vi "TestBed.vi"() -> ()   [LabVIEW 2014]
uses:
  CntrlRefs.ctl
  Modules/BusClass/Bus.lvclass
  UserEvents/clUserEventDataType.ctl
  Modules/BusClass/Bus.lvclass/Bus.ctl
  Modules/BusClass/Accessors/Write BusNumber.vi
  Modules/BusClass/Accessors/Read Test.vi
  Modules/BusClass/Accessors/Read BusNumber.vi
  <vilib>/Utility/error.llb/Error Cluster From Error Code.vi
  <vilib>/ErrorRing/Error Ring.xnode
  Modules/TestClass/Test.lvclass
  Queue/Queue.lvlib
  <userlib>/NIST/NISTErrorLib/NISTErrorLib.lvlib
  Modules/Sync/SyncModule/SyncModule.lvlib
  Modules/FGen/FgenModule/FgenModule.lvlib
  Modules/Digitizer/DigitizerModule/DigitizerModule.lvlib
  Modules/Sensor/SensorModule/SensorModule.lvlib
  Modules/Analysis/AnalysisModule/AnalysisModule.lvlib
  LV_Ini/Ini_lib.lvlib
panel:
  in  "rngDigitizer":u16(ring)=2 items=["IVI Digitizer", "Analyse Waveforms", "Debug", "Ni DaqMx Digitizer", "PMU Cal", "(obsolete)", "Simulation"]
  in  "rngFgen":u16(ring)=7 items=["DaqMx_Single", "Single_AM", "None", "Agilent IVI FGen", "IVI Dual FGens", "IVI FGen", "Debug", "Pxi6733_Sine", "Pxi6733 Sine Standalone", "PMU Cal", "Test"]
  in  "rngSync":u16(ring)=2 items=["Local", "NI PXI 6682", "6683H class Dyn3", "Debug", "Dyn3 Digitizer", "Dyn3 PMU Cal", "HIL_Sync", "Legacy", "PXI Multi"]
  in  "btnRunScript":bool
  in  "btnClearStatus":bool
  out "Status Log":string
  in  "ModuleList":string[](array[string])=["Sync", "FGen", "Digitizer"]
  in  "btnStop":bool
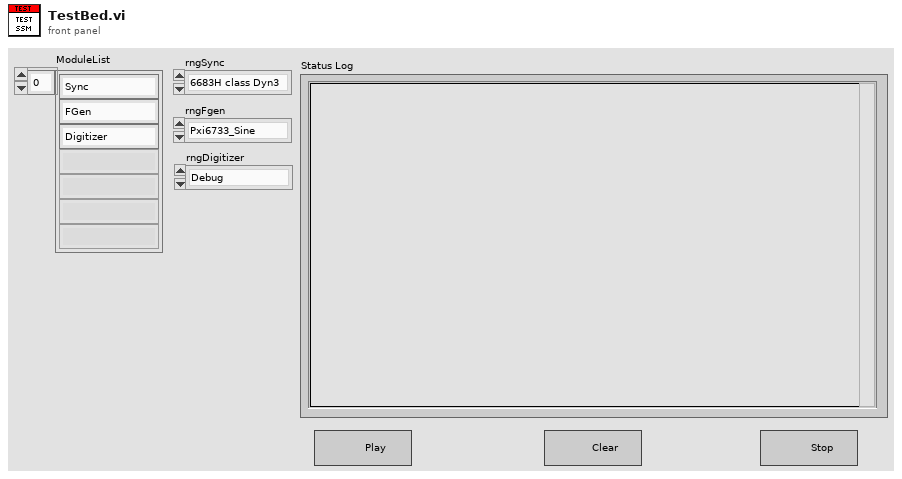
[diagram p1: front panel]
types:
  T1 = typedef "CntrlRefs.ctl" = cluster{"rngFGen":refnum<vi>, "rngDigitizer":refnum<vi>, "rngAnalysis":refnum<vi>, "rngSync":refnum<vi>, "btnHideMods":refnum<vi>, "rngSensor":refnum<vi>}
  T2 = typedef "SyncModule.lvlib/clBroadcastEvents.ctl" = cluster{"DidInit":refnum<user-event>, "StatusUpdate":refnum<user-event>, "ErrorReport":refnum<user-event>, "DidStop":refnum<user-event>, "PathToINI":refnum<user-event>, "TriggerTime":refnum<user-event>, "LockStatus":refnum<user-event>}
  T3 = typedef "FgenModule.lvlib/clBroadcastEvents.ctl" = cluster{"DidInit":refnum<user-event>, "StatusUpdate":refnum<user-event>, "ErrorReport":refnum<user-event>, "DidStop":refnum<user-event>, "PathToINI":refnum<user-event>, "Channels":refnum<user-event>, "Function":refnum<user-event>, "Waveforms":refnum<user-event>, "Triggers":refnum<user-event>}
  T4 = typedef "DigitizerModule.lvlib/clBroadcastEvents.ctl" = cluster{"DidInit":refnum<user-event>, "StatusUpdate":refnum<user-event>, "ErrorReport":refnum<user-event>, "DidStop":refnum<user-event>, "PathToINI":refnum<user-event>, "Channels":refnum<user-event>, "Acq":refnum<user-event>, "Trigger":refnum<user-event>, "Waveforms":refnum<user-event>}
  T5 = typedef "SensorModule.lvlib/clBroadcastEvents.ctl" = cluster{"DidInit":refnum<user-event>, "StatusUpdate":refnum<user-event>, "ErrorReport":refnum<user-event>, "DidStop":refnum<user-event>, "PathToINI":refnum<user-event>, "SensorReport":refnum<user-event>, "SensorConfig":refnum<user-event>}
  T6 = typedef "AnalysisModule.lvlib/clBroadcastEvents.ctl" = cluster{"DidInit":refnum<user-event>, "StatusUpdate":refnum<user-event>, "ErrorReport":refnum<user-event>, "DidStop":refnum<user-event>, "PathToINI":refnum<user-event>, "Config":refnum<user-event>, "ResultReport":refnum<user-event>}
  T7 = typedef "clUserEvents.ctl" = cluster{"StopEvent":refnum<user-event>, "CreateBus":refnum<user-event>, "UpdateEvents":refnum<user-event>}
  T8 = typedef "clUserEventDataType.ctl" = cluster{"Data":variant}
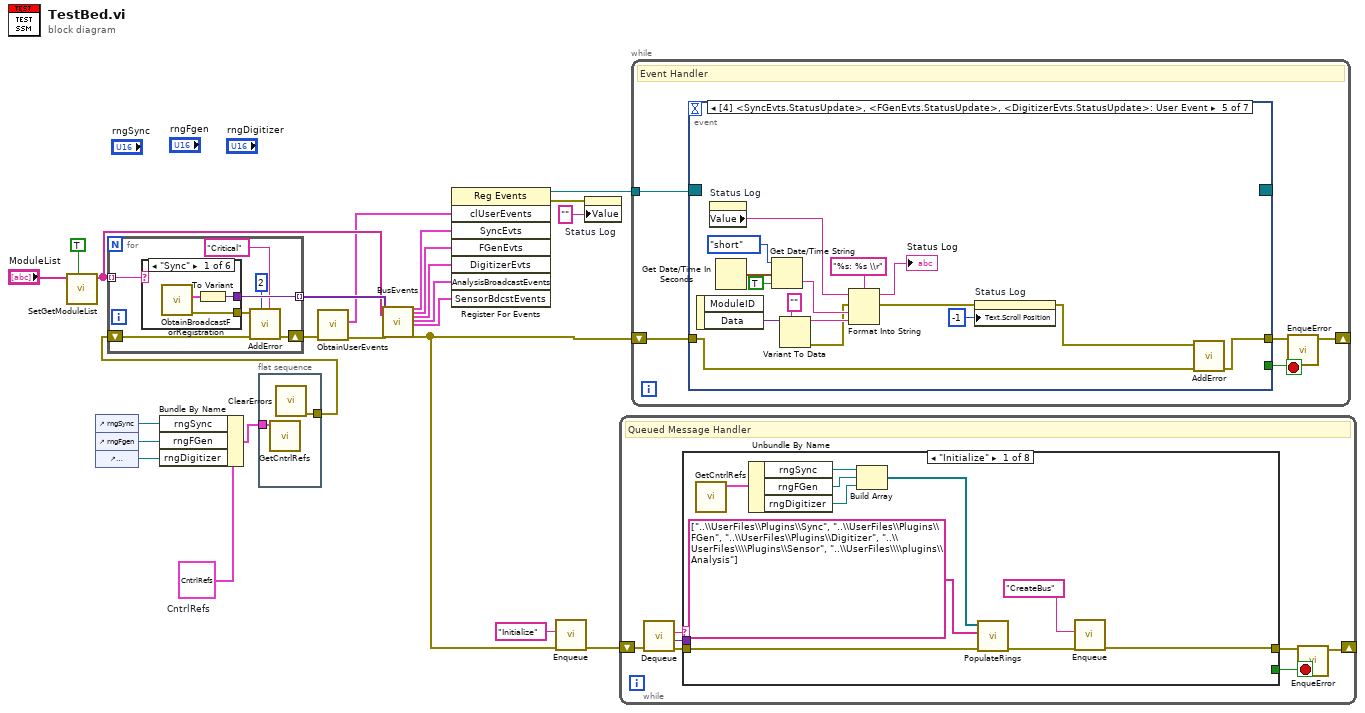
[diagram p0: block diagram]
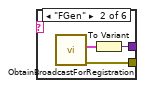
[diagram p2: hidden frame]
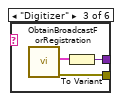
[diagram p3: hidden frame]
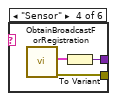
[diagram p4: hidden frame]
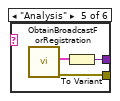
[diagram p5: hidden frame]
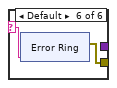
[diagram p6: hidden frame]
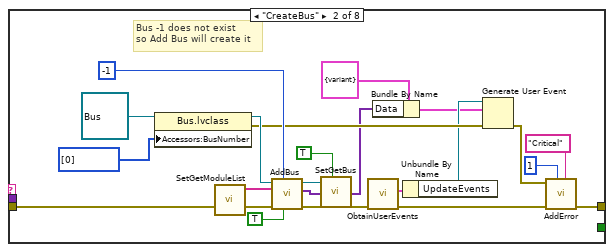
[diagram p7: hidden frame]
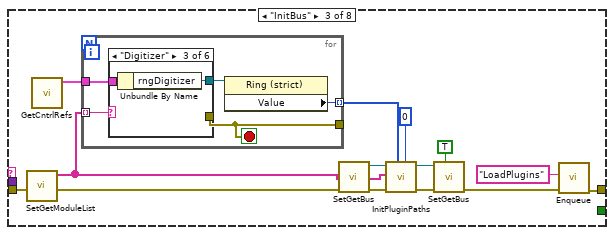
[diagram p8: hidden frame]
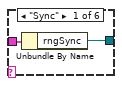
[diagram p9: hidden frame]
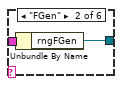
[diagram p10: hidden frame]
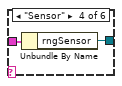
[diagram p11: hidden frame]
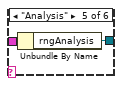
[diagram p12: hidden frame]
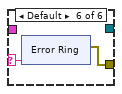
[diagram p13: hidden frame]
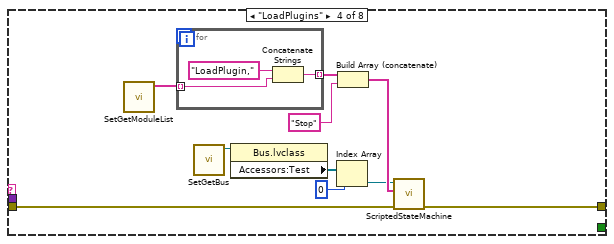
[diagram p14: hidden frame]
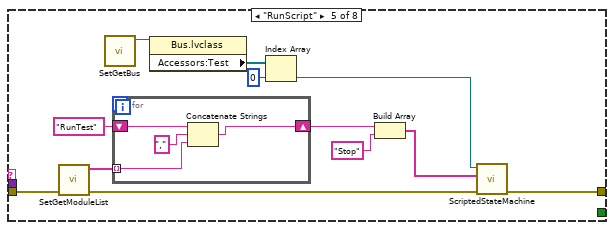
[diagram p15: hidden frame]
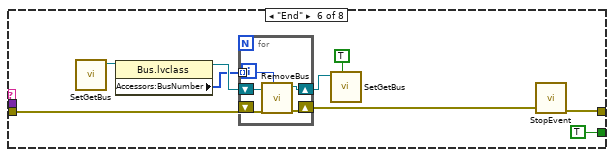
[diagram p16: hidden frame]
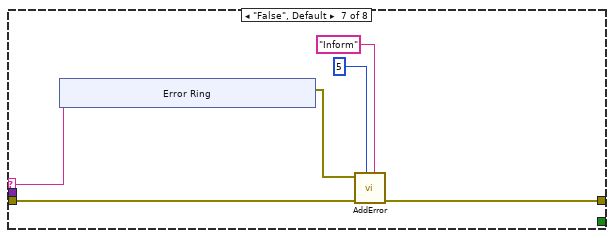
[diagram p17: hidden frame]
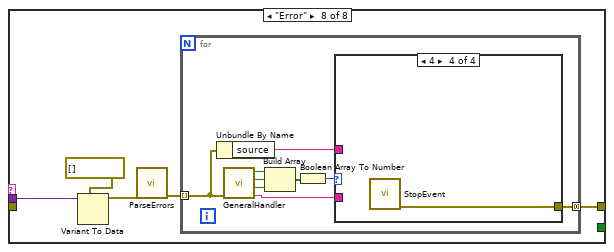
[diagram p18: hidden frame]
diagram:
  w6 = T1 {"rngFGen"=refnum, "rngDigitizer"=refnum, "rngAnalysis"=refnum, "rngSync"=refnum, "btnHideMods"=refnum, "rngSensor"=refnum}  # CntrlRefs
  n1 = call "SetGetModuleList.vi"("Set? (f)"=TRUE, "ModuleList"="ModuleList") -> ("ModuleList"=w19:string[])  [unwired: 9 in]
  n2 = control-ref of="rngSync"() -> (w5:refnum<vi>)
  n3 = control-ref of="rngFgen"() -> (w2:refnum<vi>)
  n4 = control-ref of="rngDigitizer"() -> (w1:refnum<vi>)
  n5 = for {
    shift-right: [w30] -> w9
    shift-left: w3 -> [w29]
    tunnel: [w28] -> w20 mode=indexing
    tunnel: w19 -> [w25] mode=indexing
    n6 = case shown="\"Sync\"" w25 {
      selector: w25 -> [_ _ _ _ _ w47]
      tunnel: [w33 w36 w39 w42 w45 _] -> w28
      tunnel: [w32 w37 w40 w43 w46 w48] -> w31
      frame "Sync" {
        n7 = call "ObtainBroadcastForRegistration.vi"() -> ("error out"=w32:errorcluster, "SyncBroadcastEvents"=w34:T2)  [unwired: 10 in]
        n8 = To Variant(anything=w34) -> (Variant=w33:variant)
      }
      frame "FGen" {
        n9 = call "ObtainBroadcastForRegistration.vi"() -> ("error out"=w37:errorcluster, "clBroadcastEvents"=w35:T3)  [unwired: 10 in]
        n10 = To Variant(anything=w35) -> (Variant=w36:variant)
      }
      frame "Digitizer" {
        n11 = call "ObtainBroadcastForRegistration.vi"() -> ("error out"=w40:errorcluster, "clDigitizerBdcstEvents"=w38:T4)  [unwired: 10 in]
        n12 = To Variant(anything=w38) -> (Variant=w39:variant)
      }
      frame "Sensor" {
        n13 = call "ObtainBroadcastForRegistration.vi"() -> ("error out"=w43:errorcluster, "SensorBdcstEvents"=w41:T5)  [unwired: 10 in]
        n14 = To Variant(anything=w41) -> (Variant=w42:variant)
      }
      frame "Analysis" {
        n15 = call "ObtainBroadcastForRegistration.vi"() -> ("error out"=w46:errorcluster, "AnalysisBroadcastEvents"=w44:T6)  [unwired: 10 in]
        n16 = To Variant(anything=w44) -> (Variant=w45:variant)
      }
      frame Default {
        n17 = xnode "Error Ring"("parameter 0"=w47) -> ("error out"=w48:errorcluster)
      }
    }
    n18 = call <userlib>:"AddError.vi"("Severity"="Critical", "Priority"=u8 2, "ErrorArray"=w29, "error in (no error)"=w31) -> ("ErrorArray"=w30:errorcluster[])  [unwired: 6 in, 1 out]
  }
  n19 = Bundle By Name(cluster=w6, "rngSync"=w5, "rngFGen"=w2, "rngDigitizer"=w1) -> (w4:T1)
  n20 = flat-sequence {
    tunnel: w4 -> [w57]
    tunnel: [w56] -> w3
    frame #0 {
      n21 = call "GetCntrlRefs.vi"("CntrlRefs"=w57) -> ()  [unwired: 10 in, 1 out]
      n22 = call <userlib>:"ClearErrors.vi"() -> ("ErrorArray"=w56:errorcluster[])  [unwired: 11 in]
    }
  }
  n23 = call "ObtainUserEvents.vi"("ErrorArray"=w9) -> ("ErrorArray"=w8:errorcluster[], "clUserEvents"=w7:T7)  [unwired: 9 in]
  n24 = call "BusEvents.vi"("EventArray"=w20, "Error in"=w8, "ModuleList"=w19) -> ("SyncEvts"=w12:T2, "FGenEvts"=w17:T3, "DigitizerEvts"=w16:T4, "AnalysisBroadcastEvents"=w15:T6, "SensorBdcstEvents"=w14:T5, "Error out"=w13:errorcluster[])  [unwired: 18 in, 1 out]
  n25 = register-events(w7, w12, w17, w16, w15, w14) -> (reference out=w18:refnum<event-registration>, error out=w11:errorcluster)  [unwired: 2 in]
  n26 = call "Enqueue.vi"("ErrorArray"=w13, "Message"="Initialize") -> ("ErrorArray"=w23:errorcluster[])  [unwired: 9 in]
  n27 = property on="Status Log" class="Str"(error in=w11, "Value"="") -> ()  [unwired: 1 in, 2 out]
  n28 = while {
    shift-right: [w59] -> _
    shift-left: w23 -> [w64]
    stop <- w58 stop-if-true
    # "Queued Message Handler"
    n29 = call "Dequeue.vi"("ErrorArray"=w64) -> ("ErrorArray"=w61:errorcluster[], "Message Data"=w62:variant, "Message"=w63:string)  [unwired: 8 in]
    n30 = case shown="\"Initialize\"" w63 {
      selector: w63 -> [_ _ _ _ _ _ w178 _]
      tunnel: w62 -> [_ _ _ _ _ _ _ w187]
      tunnel: w61 -> [w72 w91 w106 w133 w145 w162 w177 _]
      tunnel: [w67 w86 w100 w132 w144 w160 w173 w186] -> w60
      tunnel: [_ _ _ _ _ TRUE _ _] -> w58
      frame "Initialize" {
        n31 = call "GetCntrlRefs.vi"() -> ("CntrlRefs"=w74:T1)  [unwired: 11 in]
        n32 = Unbundle By Name(w74) -> ("rngSync"=w73:refnum<vi>, "rngFGen"=w66:refnum<vi>, "rngDigitizer"=w65:refnum<vi>)
        n33 = Build Array(w73, w66, w65) -> (w71:refnum<vi>[])
        n34 = call "PopulateRings.vi"("ErrorArray In"=w72, "RelativePathToIniArray"=string[] ["..\\UserFiles\\Plugins\\Sync", "..\\UserFiles\\Plugins\\FGen", "..\\UserFiles\\Plugins\\Digitizer", "..\\UserFiles\\\\Plugins\\Sensor", "..\\UserFiles\\\\plugins\\Analysis"], "RingRefArray"=w71) -> ("ErrorArray Out"=w69:errorcluster[])  [unwired: 7 in, 1 out]
        n35 = call "Enqueue.vi"("ErrorArray"=w69, "Message"="CreateBus") -> ("ErrorArray"=w67:errorcluster[])  [unwired: 9 in]
      }
      frame "CreateBus" {
        # "Bus -1 does not exist\nso Add Bus will create it"
        n36 = property class="Bus.lvclass"(reference=refnum<class "Bus.lvclass"> refnum ("Bus.lvclass"), "Accessors:BusNumber"=i32[] [0] ("BusNumber")) -> (reference out=w92:refnum<class "Bus.lvclass">, error out=w82:errorcluster)  [unwired: 1 in]
        n37 = call "SetGetModuleList.vi"() -> ("ModuleList"=w95:string[])  [unwired: 11 in]
        n38 = call "AddBus.vi"("ShowPanel? (f)"=TRUE, "BusNumber"=-1, "ErrorIn"=w91, "ModuleList"=w95, "Bus.lvclass"=w92) -> ("ErrorOut"=w81:errorcluster[], "UsrEvents"=w76:variant[], "Bus.lvclass"=w88:refnum<class "Bus.lvclass">)  [unwired: 4 in]
        n39 = call "SetGetBus.vi"("Set (f)"=TRUE, "Bus.lvclass"=w88) -> ()  [unwired: 9 in, 1 out]
        n40 = call "ObtainUserEvents.vi"("ErrorArray"=w81) -> ("ErrorArray"=w80:errorcluster[], "clUserEvents"=w79:T7)  [unwired: 9 in]
        n41 = Bundle By Name(cluster=T8 {"Data"=variant} ("clUserEventData"), "Data"=w76) -> (w75:T8)
        n42 = Unbundle By Name(w79) -> ("UpdateEvents"=w78:refnum<user-event>)
        n43 = Generate User Event(user event=w78, event data cluster=w75, error in=w82) -> (error out=w85:errorcluster)  [unwired: 1 in, 1 out]
        n44 = call <userlib>:"AddError.vi"("Severity"="Critical", "Priority"=u8 1, "ErrorArray"=w80, "error in (no error)"=w85) -> ("ErrorArray"=w86:errorcluster[])  [unwired: 6 in, 1 out]
      }
      frame "InitBus" {
        n45 = call "SetGetModuleList.vi"() -> ("ModuleList"=w97:string[])  [unwired: 11 in]
        n46 = call "GetCntrlRefs.vi"() -> ("CntrlRefs"=w98:T1)  [unwired: 11 in]
        n47 = for {
          tunnel: w97 -> [w111] mode=indexing
          tunnel: w98 -> [w110]
          tunnel: [w108] -> w96 mode=indexing
          tunnel: [w107] -> _
          stop <- w107 stop-if-true
          n48 = case shown="\"Digitizer\"" w111 {
            selector: w111 -> [_ _ _ _ _ w123]
            tunnel: w110 -> [w113 w115 w117 w119 w121 _]
            tunnel: [w112 w114 w116 w118 w120 _] -> w109
            tunnel: [_ _ _ _ _ w122] -> w107
            frame "Sync" {
              n49 = Unbundle By Name(w113) -> ("rngSync"=w112:refnum<vi>)
            }
            frame "FGen" {
              n50 = Unbundle By Name(w115) -> ("rngFGen"=w114:refnum<vi>)
            }
            frame "Digitizer" {
              n51 = Unbundle By Name(w117) -> ("rngDigitizer"=w116:refnum<vi>)
            }
            frame "Sensor" {
              n52 = Unbundle By Name(w119) -> ("rngSensor"=w118:refnum<vi>)
            }
            frame "Analysis" {
              n53 = Unbundle By Name(w121) -> ("rngAnalysis"=w120:refnum<vi>)
            }
            frame Default {
              n54 = xnode "Error Ring"("parameter 0"=w123) -> ("error out"=w122:errorcluster)
            }
          }
          n55 = property class="Ring (strict)"(reference=w109) -> ("Value"=w108:u16)  [unwired: 1 in, 2 out]
        }
        n56 = call "SetGetBus.vi"() -> ("Bus.lvclass"=w105:refnum<class "Bus.lvclass">)  [unwired: 11 in]
        n57 = call "InitPluginPaths.vi"("BusIndex"=0, "PluginIndex"=w96, "Error In"=w106, "Modules"=w97, "Bus in"=w105) -> ("Error Out"=w101:errorcluster[], "Bus out"=w104:refnum<class "Bus.lvclass">)  [unwired: 5 in]
        n58 = call "SetGetBus.vi"("Set (f)"=TRUE, "Bus.lvclass"=w104) -> ()  [unwired: 9 in, 1 out]
        n59 = call "Enqueue.vi"("ErrorArray"=w101, "Message"="LoadPlugins") -> ("ErrorArray"=w100:errorcluster[])  [unwired: 9 in]
      }
      frame "LoadPlugins" {
        n60 = call "SetGetModuleList.vi"() -> ("ModuleList"=w131:string[])  [unwired: 11 in]
        n61 = for {
          tunnel: w131 -> [w142] mode=indexing
          tunnel: [w141] -> w134 mode=indexing
          n62 = Concatenate Strings("LoadPlugin," ("string"), w142) -> (w141:string)
        }
        n63 = call "SetGetBus.vi"() -> ("Bus.lvclass"=w136:refnum<class "Bus.lvclass">)  [unwired: 11 in]
        n64 = property class="Bus.lvclass"(reference=w136) -> ("Accessors:Test"=w137:refnum<class "Test.lvclass">[])  [unwired: 1 in, 2 out]
        n65 = Index Array(array=w137, index=0) -> (element=w139:refnum<class "Test.lvclass">)
        n66 = Build Array (concatenate)(w134, "Stop" ("string")) -> (w140:string[])
        n67 = call "ScriptedStateMachine.vi"("ErrorArray"=w133, "script"=w140, "Test.lvclass"=w139) -> ("ErrorArray"=w132:errorcluster[])  [unwired: 6 in, 2 out]
      }
      frame "RunScript" {
        n68 = call "SetGetModuleList.vi"() -> ("ModuleList"=w148:string[])  [unwired: 11 in]
        n69 = call "SetGetBus.vi"() -> ("Bus.lvclass"=w154:refnum<class "Bus.lvclass">)  [unwired: 11 in]
        n70 = for {
          tunnel: w148 -> [w156] mode=indexing
          shift-right: [w155] -> w149
          shift-left: "RunTest" -> [w158]
          n71 = Concatenate Strings(w158, ",", w156) -> (w155:string)
        }
        n72 = property class="Bus.lvclass"(reference=w154) -> ("Accessors:Test"=w153:refnum<class "Test.lvclass">[])  [unwired: 1 in, 2 out]
        n73 = Index Array(array=w153, index=0) -> (element=w151:refnum<class "Test.lvclass">)
        n74 = Build Array(w149, "Stop") -> (w147:string[])
        n75 = call "ScriptedStateMachine.vi"("ErrorArray"=w145, "script"=w147, "Test.lvclass"=w151) -> ("ErrorArray"=w144:errorcluster[])  [unwired: 6 in, 2 out]
      }
      frame "End" {
        n76 = call "SetGetBus.vi"() -> ("Bus.lvclass"=w165:refnum<class "Bus.lvclass">)  [unwired: 11 in]
        n77 = property class="Bus.lvclass"(reference=w165) -> (reference out=w167:refnum<class "Bus.lvclass">, "Accessors:BusNumber"=w166:i32[])  [unwired: 1 in, 1 out]
        n78 = for {
          tunnel: w166 -> [w169] mode=indexing
          shift-right: [w170] -> w159
          shift-left: w162 -> [w171]
          shift-right: [w168] -> w164
          shift-left: w167 -> [w172]
          n79 = call "RemoveBus.vi"("BusNumber"=w169, "ErrorIn"=w171, "Bus.lvclass"=w172) -> ("ErrorOut"=w170:errorcluster[], "Bus.lvclass"=w168:refnum<class "Bus.lvclass">)  [unwired: 7 in]
        }
        n80 = call "SetGetBus.vi"("Set (f)"=TRUE, "Bus.lvclass"=w164) -> ()  [unwired: 9 in, 1 out]
        n81 = call "StopEvent.vi"("ErrorArray"=w159) -> ("ErrorArray"=w160:errorcluster[])  [unwired: 10 in]
      }
      frame "False", Default {
        n82 = xnode "Error Ring"("parameter 0"=w178) -> ("error out"=w176:errorcluster)
        n83 = call <userlib>:"AddError.vi"("Severity"="Inform", "Priority"=u8 5, "ErrorArray"=w177, "error in (no error)"=w176) -> ("ErrorArray"=w173:errorcluster[])  [unwired: 6 in, 1 out]
      }
      frame "Error" {
        n84 = Variant To Data(type=errorcluster[] [] ("ErrorArray"), Variant=w187) -> (data=w189:errorcluster[])  [unwired: 1 in, 1 out]
        n85 = call <userlib>:"ParseErrors.vi"("ErrorArray"=w189) -> ("ErrorArray"=w190:errorcluster[])  [unwired: 8 in, 2 out]
        n86 = for {
          tunnel: w190 -> [w199] mode=indexing
          tunnel: [w191] -> w186 mode=concatenating
          n87 = Unbundle By Name(w199) -> ("source"=w193:string)
          n88 = call <userlib>:"GeneralHandler.vi"("error in (no error)"=w199) -> ("Severity"=w192:string, "Stop"=w196:bool, "Abort"=w197:bool, "Continue"=w198:bool)  [unwired: 7 in]
          n89 = Build Array(w198, w197, w196) -> (w195:bool[])
          n90 = Boolean Array To Number(Boolean array=w195) -> (number=w194:u32)
          n91 = case shown="4" w194 {
            tunnel: w193 -> [_ _ _ _]
            tunnel: w192 -> [_ w200 _ _]
            tunnel: [_ _ w201 w207] -> w191
            frame 0, Default {
              # "No Dialog"
            }
            frame 1 {
              # "Continue"
              n92 = case shown="\"Log\"" w200 {
                frame Default {
                  # "Continue operation"
                }
                frame "Log" {
                  # "TODO: if your program\nhas a log file.  Write to \nit here."
                  # "Write to log file"
                }
              }
            }
            frame 2 {
              # "Abort Button Pressed"
              n93 = call "ObtainQueue.vi"() -> ("ErrorArray"=w204:errorcluster[], "QueueRef"=w206:refnum<queue>)  [unwired: 10 in]
              n94 = Flush Queue(queue=w206) -> (error out=w205:errorcluster)  [unwired: 1 in, 2 out]
              n95 = call <userlib>:"AddError.vi"("Severity"="Critical", "Priority"=u8 1, "ErrorArray"=w204, "error in (no error)"=w205) -> ("ErrorArray"=w201:errorcluster[])  [unwired: 6 in, 1 out]
            }
            frame 4 {
              n96 = call "StopEvent.vi"() -> ("ErrorArray"=w207:errorcluster[])  [unwired: 11 in]
            }
          }
        }
      }
    }
    n97 = call "EnqueError.vi"("ErrorArray"=w60) -> ("ErrorArray 2"=w59:errorcluster[])  [unwired: 10 in]
  }
  n98 = while {
    shift-right: [w211] -> _
    shift-left: w13 -> [w210]
    tunnel: w18 -> [w208]
    stop <- w209 stop-if-true
    # "Event Handler"
    n99 = event shown="[4] <SyncEvts.StatusUpdate>, <FGenEvts.StatusUpdate>, <DigitizerEvts.StatusUpdate>: User Event" {
      selector: w208 -> [_ w232 _ _ _ _ _]
      dyn-events: [_ w225 _ _ _ _ _] -> _
      timeout: _ -> [_ _ _ _ _ _ _]
      tunnel: [w213 w234 w236 w240 w244 w259 w279] -> w212
      tunnel: w210 -> [w214 w222 w238 w240 w248 w264 w280]
      tunnel: [_ _ _ _ _ _ TRUE] -> w209
      event "btnStop": Value Change {
        n100 = event-data() -> ()  [unwired: 1 in, 1 out]
        n101 = call "Enqueue.vi"("Priority (F)"=TRUE, "ErrorArray"=w214, "Message"="End") -> ("ErrorArray"=w213:errorcluster[])  [unwired: 8 in]
      }
      event User Event {
        n102 = event-data() -> ("Data"=w217:variant)  [unwired: 1 in]
        n103 = Variant To Data(type=variant[] [], Variant=w217) -> (data=w223:variant[], error out=w220:errorcluster)  [unwired: 1 in]
        n104 = call <userlib>:"AddError.vi"("Severity"="Critical", "Priority"=u8 1, "ErrorArray"=w222, "error in (no error)"=w220) -> ("ErrorArray"=w221:errorcluster[])  [unwired: 6 in, 1 out]
        n105 = call "SetGetModuleList.vi"() -> ("ModuleList"=w233:string[])  [unwired: 11 in]
        n106 = call "BusEvents.vi"("EventArray"=w223, "Error in"=w221, "ModuleList"=w233) -> ("SyncEvts"=w231:T2, "FGenEvts"=w230:T3, "DigitizerEvts"=w229:T4, "AnalysisBroadcastEvents"=w228:T6, "SensorBdcstEvents"=w227:T5, "Error out"=w226:errorcluster[])  [unwired: 18 in, 1 out]
        n107 = register-events(reference=w232, w231, w230, w229, w228, w227) -> (reference out=w225:refnum<event-registration>)  [unwired: 2 in, 1 out]
        n108 = call "Enqueue.vi"("ErrorArray"=w226, "Message"="InitBus") -> ("ErrorArray"=w234:errorcluster[])  [unwired: 9 in]
      }
      event "btnRunScript": Value Change {
        n109 = event-data() -> ()  [unwired: 1 in, 1 out]
        n110 = call "Enqueue.vi"("ErrorArray"=w238, "Message"="RunScript") -> ("ErrorArray"=w236:errorcluster[])  [unwired: 9 in]
      }
      event "btnClearStatus": Value Change {
        n111 = event-data() -> ()  [unwired: 1 in, 1 out]
        n112 = property on="Status Log" class="Str"("Value"="") -> ()  [unwired: 2 in, 2 out]
      }
      event User Event {
        n113 = event-data() -> ("Data"=w253:variant)  [unwired: 1 in, 1 out]
        n114 = property on="Status Log" class="Str"() -> ("Value"=w247:string)  [unwired: 2 in, 2 out]
        n115 = Get Date/Time In Seconds() -> (seconds since 1Jan1904=w254:timestamp)
        n116 = Get Date/Time String(date format (0)=enum16{"short", "long", "abbreviated"}."short", seconds (now)=w254, want seconds? (F)=TRUE) -> (time string=w249:string)  [unwired: 1 out]
        n117 = Variant To Data(type="", Variant=w253) -> (data=w251:string, error out=w245:errorcluster)  [unwired: 1 in]
        n118 = Format Into String(format string="%s: %s \\r", initial string=w247, error in=w245, w249, w251) -> (resulting string=→"Status Log":string, error out=w243:errorcluster)
        n119 = property on="Status Log" class="Str"(error in=w243, "Text.Scroll Position"=-1) -> (error out=w242:errorcluster)  [unwired: 1 in, 1 out]
        n120 = call <userlib>:"AddError.vi"("ErrorArray"=w248, "error in (no error)"=w242) -> ("ErrorArray"=w244:errorcluster[])  [unwired: 8 in, 1 out]
      }
      event User Event {
        n121 = event-data() -> ("ModuleID"=w263:i32, "Data"=w262:variant)  [unwired: 1 in]
        n122 = Get Date/Time In Seconds() -> (seconds since 1Jan1904=w270:timestamp)
        n123 = property on="Status Log" class="Str"() -> ("Value"=w261:string)  [unwired: 2 in, 2 out]
        n124 = Variant To Data(type=errorcluster {"status"=FALSE, "code"=0, "source"=""} ("error constant"), Variant=w262) -> (data=w274:errorcluster, error out=w275:errorcluster)  [unwired: 1 in]
        n125 = Get Date/Time String(date format (0)=enum16{"short", "long", "abbreviated"}."short", seconds (now)=w270, want seconds? (F)=TRUE) -> (time string=w267:string)  [unwired: 1 out]
        n126 = Unbundle By Name(w274) -> ("source"=w266:string)
        n127 = Merge Errors(w274, w275) -> (w273:errorcluster)
        n128 = call <userlib>:"AddError.vi"("Severity"="UserOption", "Priority"=u8 2, "ErrorArray"=w264, "error in (no error)"=w273) -> ("ErrorArray"=w259:errorcluster[])  [unwired: 6 in, 1 out]
        n129 = Format Into String(format string="%s: Module %d:  %s \\r", initial string=w261, w267, w263, w266) -> (resulting string=w260:string, error out=w258:errorcluster)  [unwired: 1 in]
        n130 = property on="Status Log" class="Str"("Value"=w260) -> ()  [unwired: 2 in, 2 out]
        n131 = property on="Status Log" class="Str"(error in=w258, "Text.Scroll Position"=-1) -> ()  [unwired: 1 in, 2 out]
      }
      event User Event {
        n132 = event-data() -> ()  [unwired: 1 in, 1 out]
        n133 = call "Enqueue.vi"("Priority (F)"=TRUE, "ErrorArray"=w280, "Message"="End") -> ("ErrorArray"=w279:errorcluster[])  [unwired: 8 in]
      }
    }
    n134 = call "EnqueError.vi"("ErrorArray"=w212) -> ("ErrorArray 2"=w211:errorcluster[])  [unwired: 10 in]
  }
